vi "MEASURE_hysteresis_multiple_SHG gate_pmt-final.vi"() -> ()   [LabVIEW 2020]
uses:
  <vilib>/DAQmx/read.llb/DAQmx Read.vi
  <vilib>/DAQmx/read.llb/DAQmx Read (Counter U32 1Chan 1Samp).vi
  <vilib>/Analysis/baseanly.llb/Mean (DBL).vi
  <vilib>/DAQmx/create/channels.llb/DAQmx Create Channel (CI-Count Edges).vi
  <instrlib>/Keithley 24XX/Public/Data/Read (Multiple Points).vi
  <vilib>/DAQmx/miscellaneous.llb/DAQmx Fill In Error Info.vi
  <vilib>/Utility/file.llb/Write To Spreadsheet File (DBL).vi
  <instrlib>/Stanford Research 830/Stanford Research 830.lvlib
  <instrlib>/Keithley 2450/Keithley 2450.lvlib
  <resource>/objmgr/daqmx.rc
  <instrlib>/Keithley 24XX/Keithley 24XX.lvlib
  <vilib>/Analysis/NI_AALBase.lvlib
panel:
  in  "topgate-off set":dbl=-5.0
  in  "0ff set{T}/no off set[F]":bool
  out "XY Graph 4":cluster{dbl[], dbl[]}(graph)
  out "XY Graph 3":cluster{dbl[], dbl[]}(graph)
  out "back gate leaking":dbl=2.469318360898143e-10
  out "top gate voltage":dbl format="%#_13g"
  in  "Compliance  Level (1uA)":dbl=1.9999999995789155e-07
  in  "Source Mode  (0: Voltage)":u16(ring) items=["Voltage", "Current"]
  in  "Serial Configuration":T1={"Baud Rate"=9600, "Parity"=0, "Data Bits"=8, "Stop Bits"=10, "Flow Control"=0} {"Flow Control" items=["None", "XON/XOFF", "RTS/CTS", "XON/XOFF & RTS/CTS", "DTR/DSR", "XON/XOFF & DTR/DSR"]; "Stop Bits" items=["1.0"=10, "1.5"=15, "2.0"=20]; "Data Bits" items=["7"=7, "8"=8]; "Parity" items=["None", "Odd", "Even", "Mark", "Space"]; "Baud Rate" items=["300"=300, "600"=600, "1200"=1200, "2400"=2400, "4800"=4800, "9600"=9600, "19200"=19200]}
  in  "back gate address":refnum<visa-resource-name>="GPIB0::25::INSTR"
  in  "top gate thickness":dbl=10.0
  in  "back gate thickness":dbl=30.0
  in  "pure field (T)/pure doping (F)":bool
  in  "Clear Plot 2":bool
  out "XY Graph 2":cluster{dbl[], dbl[]}(graph)
  in  "accumulation":i32=80
  out "Waveform Chart 3":dbl[](graph)=[376.0, 339.0, 337.0, 347.0, 368.0, 343.0, 313.0, 342.0, 356.0, 353.0, 315.0, 360.0, 375.0, 301.0, 363.0, 324.0, 334.0, 324.0, 318.0, 329.0, 312.0, 341.0, 352.0, 336.0, 351.0, 312.0, 361.0, 339.0, 352.0, 315.0, 360.0, 366.0, 324.0, 343.0, 343.0, 330.0, 340.0, 327.0, 393.0, 330.0, 335.0, 353.0, 360.0, 347.0, 337.0, 336.0, 312.0, 331.0, 326.0, 350.0, 344.0, 328.0, 357.0, 355.0, 356.0, 331.0, 328.0, 340.0, 355.0, 387.0, 371.0, 360.0, 331.0, 339.0, 344.0, 367.0, 343.0, 360.0, 360.0, 370.0, 335.0, 366.0, 323.0, 378.0, 373.0, 358.0]
  out "Numeric":dbl=344.60526315789474
  in  "Counter Channel":tag="/Dev1/PFI0"
  in  "error in":errorcluster
  out "loop run":i32=2
  in  "loop #":i32=2
  in  "Save data or not":bool=TRUE
  in  "path (folder + filename)":string="C:\\Users\\User\\Data\\Jason\\03282019\\ pure_bottom_high_6v_rato3 with light2"
  in  "Clear Plot":bool
  out "LOCKIN Measurement":dbl=0.9110010000000001
  in  "Parameter (1: X)":u16(ring)=1 items=["X"=1, "Y"=2, "R"=3, "Theta"=4, "Channel 1"=5, "Channel 2"=6, "Aux In 1"=7, "Aux In 2"=8, "Aux In 3"=9, "Aux In 4"=10]
  out "back gate voltage":dbl format="%#_13g"
  out "top gate leaking":string="-9.306248E-12\n"
  in  "GATE STEP(mv)":i32=450
  in  "GATE Low Value (default 0)":dbl
  in  "GATE High Value":dbl=18.0
  in  "Function (0: Volts) 2":u16(ring) items=["Volts", "Current", "Resistance"]
  in  "Source Compaliance":dbl=1.000000000000001e-07
  in  "topgate address":refnum<visa-resource-name>="GPIB0::18::INSTR"
  in  "SD stabilization(S) 2":dbl=0.1 format="%#_13g"
  in  "Sine Output Amplitude (1 V) 2":dbl=0.05
  in  "GATE / SD stablization 3":dbl=0.1 format="%#_13g"
  in  "frequency":dbl=50.0 format="%#_13g"
  in  "Input Connection (0: Single-Ended Voltage)":u16(ring) items=["Single-Ended Voltage", "Differential Voltage", "1 MOhm Current Gain", "100 MOhm Current Gain"]
  in  "LOCKIN address":refnum<visa-resource-name>="GPIB0::8::INSTR"
  # "Gate2401(top) Setting"
  # "Lock-in"
  # "Gate2450(back) Setting"
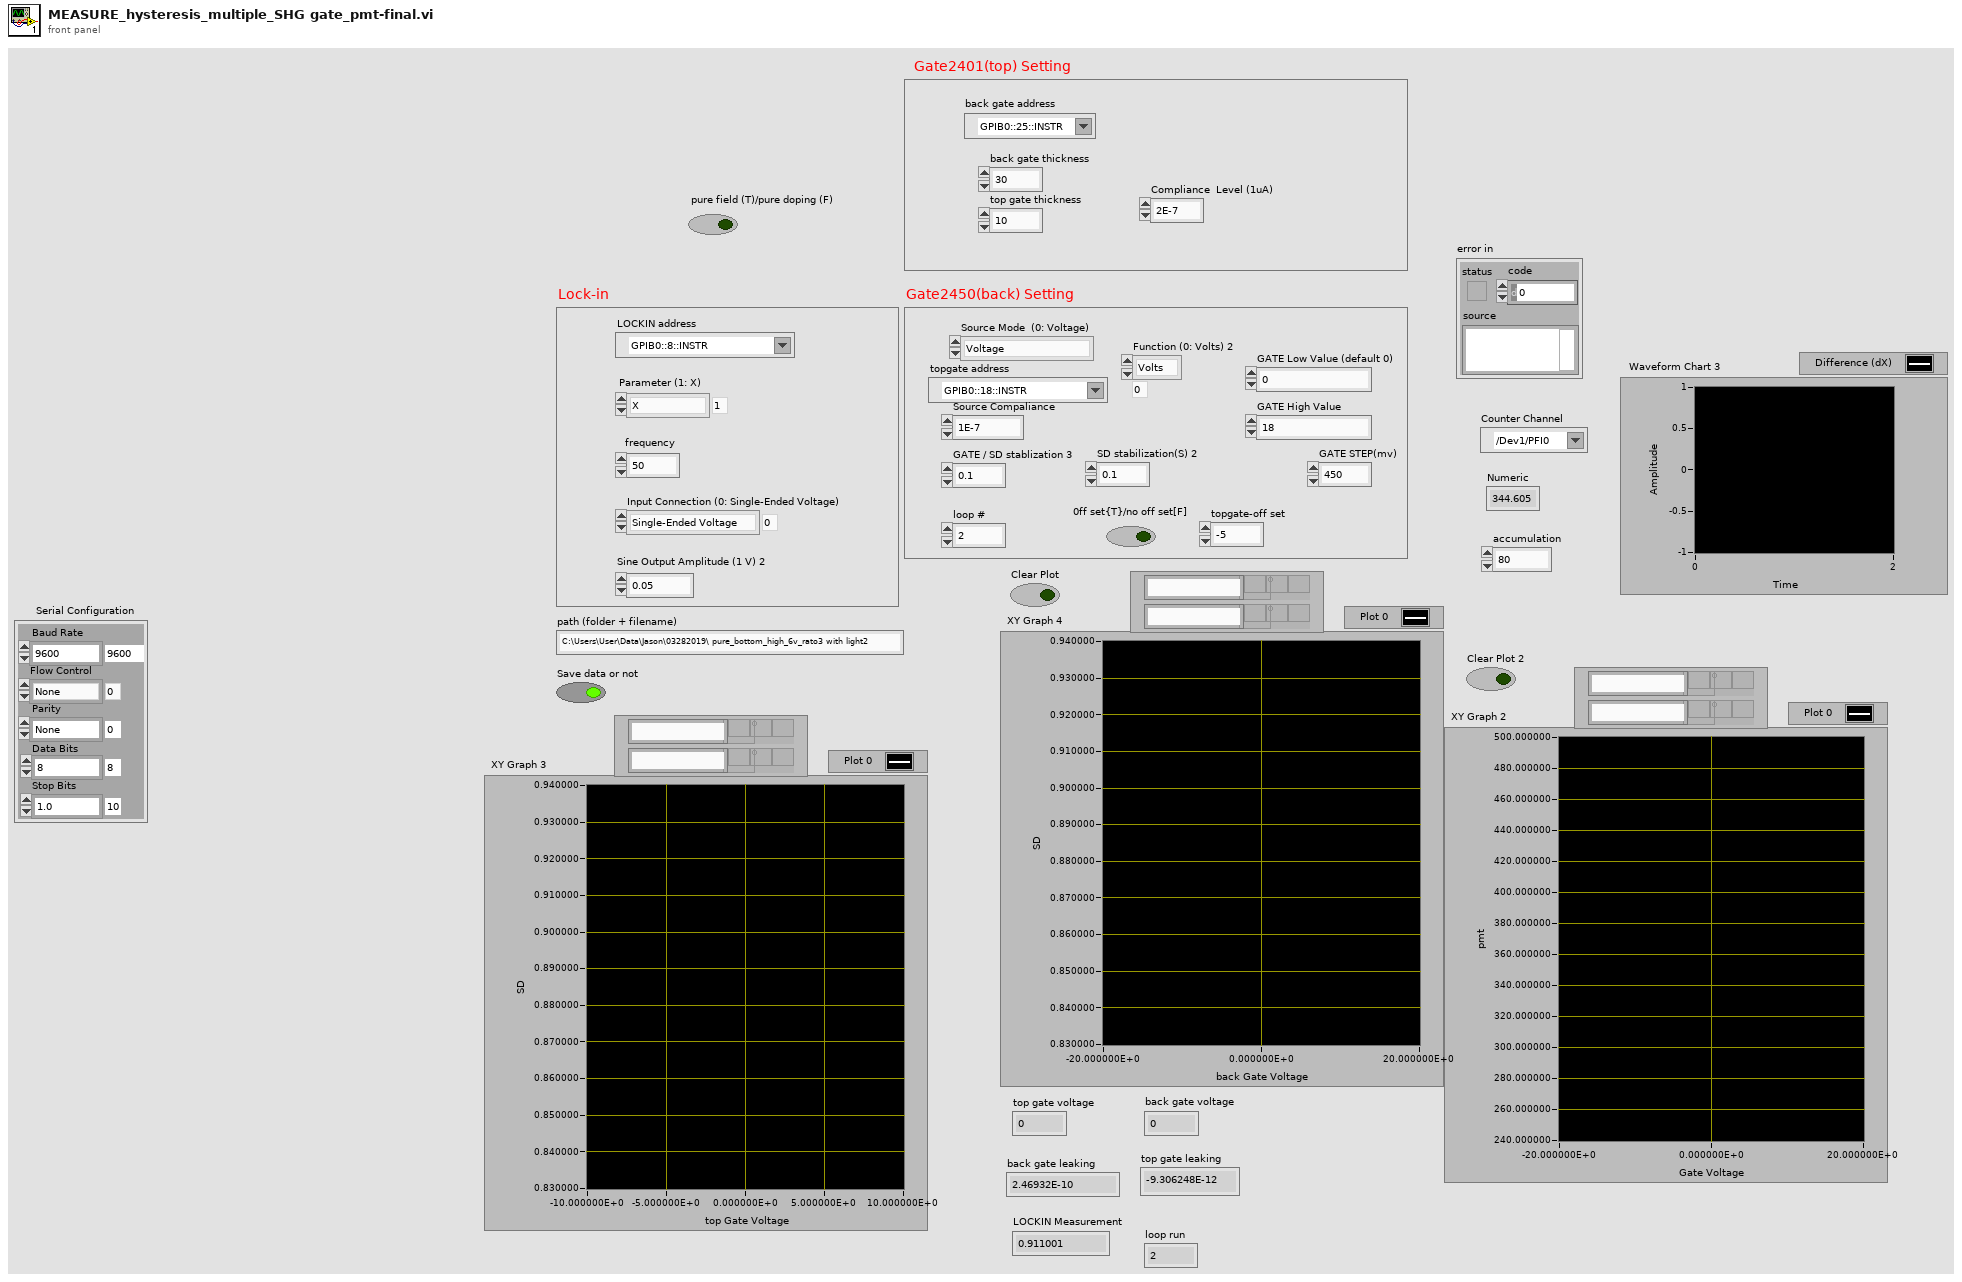
[diagram p1: front panel]
types:
  T1 = cluster{"Baud Rate":u32, "Parity":u16, "Data Bits":u16, "Stop Bits":u16, "Flow Control":u16}
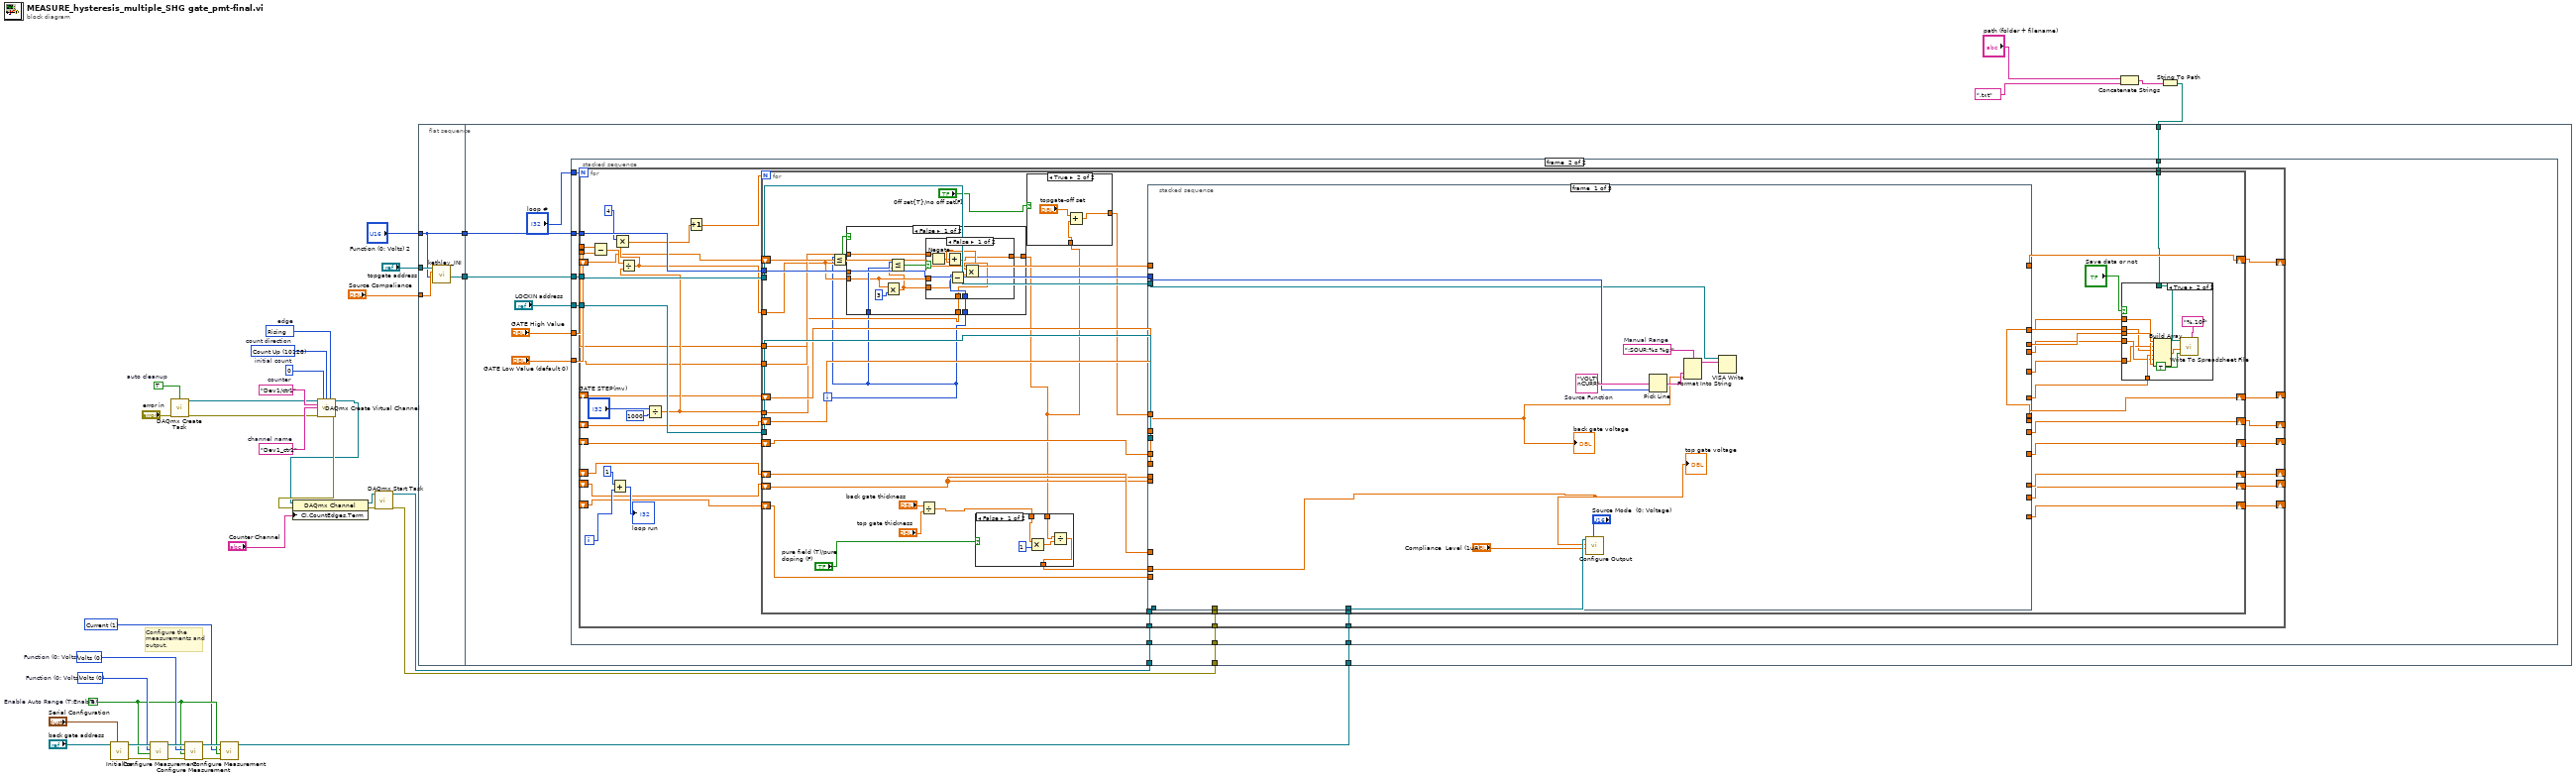
[diagram p0: block diagram]
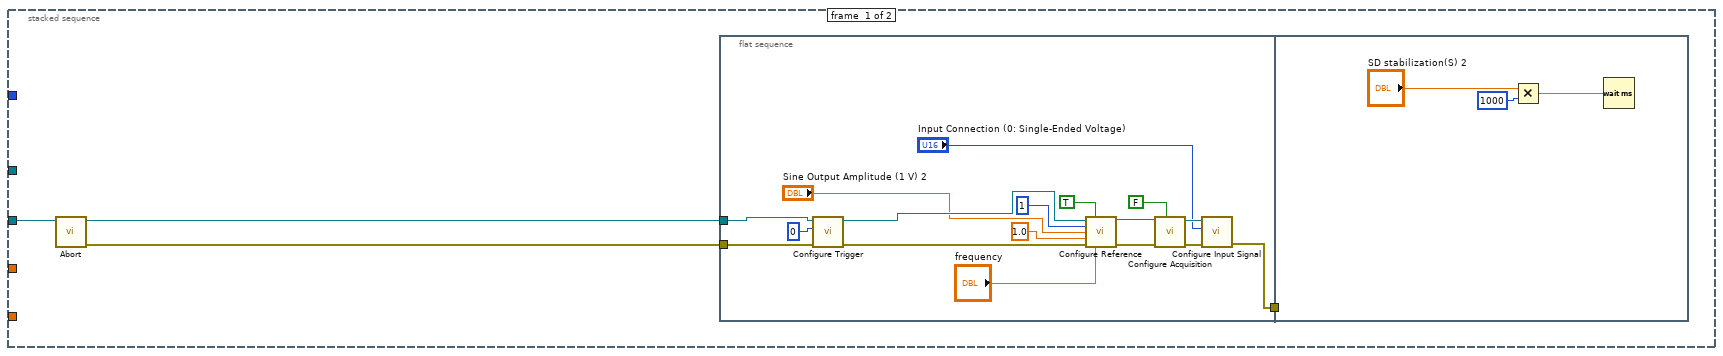
[diagram p2: hidden frame]
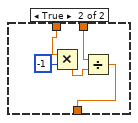
[diagram p4: hidden frame]
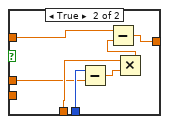
[diagram p6: hidden frame]
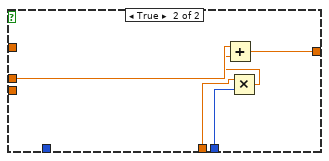
[diagram p7: hidden frame]
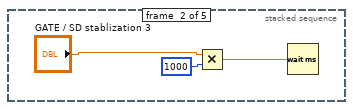
[diagram p8: hidden frame]
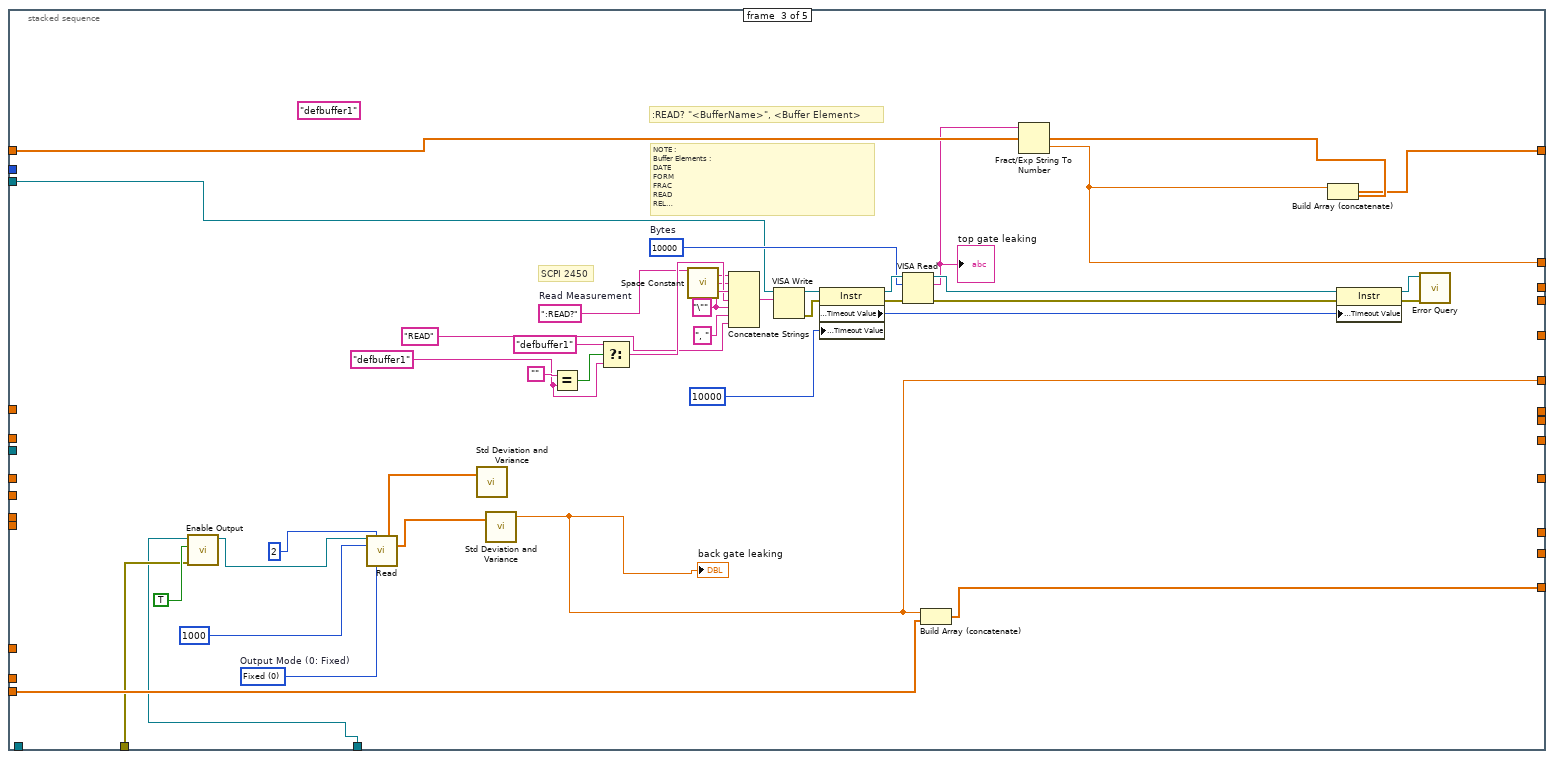
[diagram p9: hidden frame]
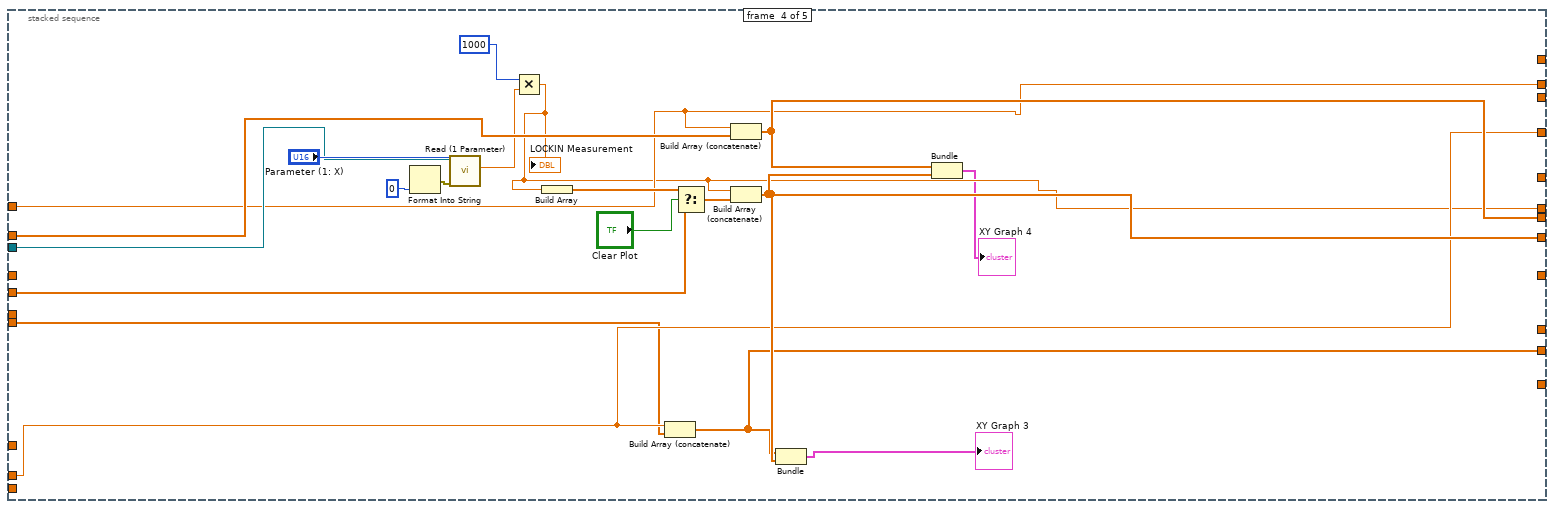
[diagram p10: hidden frame]
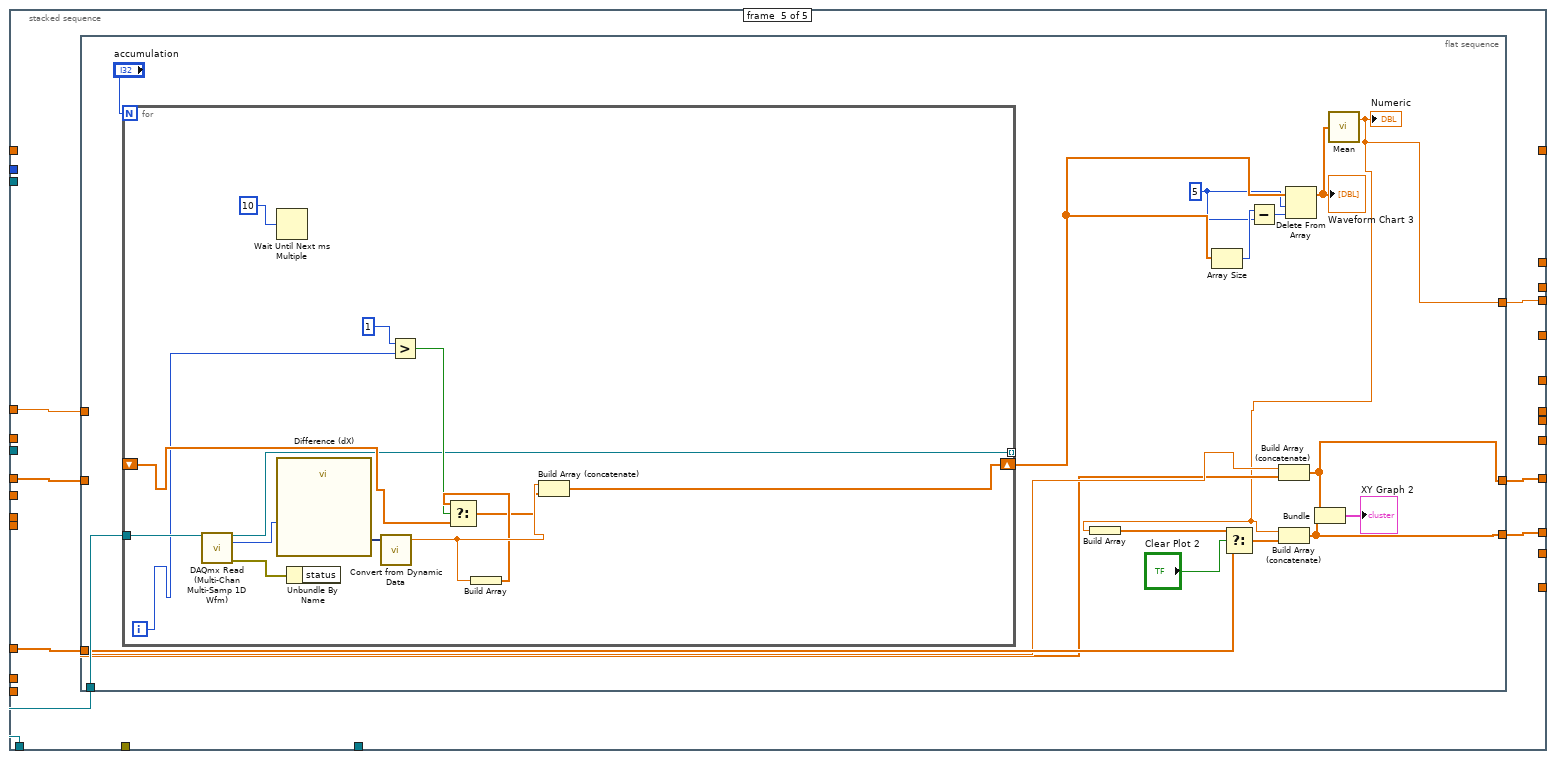
[diagram p11: hidden frame]
diagram:
  w3 = u16 1 items=["Volts", "Current", "Resistance"] ("Function (0: Volts)")
  w4 = TRUE  # Enable Auto Range (T:Enable)
  w7 = u16 0 items=["Volts", "Current", "Resistance"]  # Function (0: Volts)
  w8 = u16 0 items=["Volts", "Current", "Resistance"]  # Function (0: Volts)
  w27 = 10280 items=["Rising"=10280, "Falling"=10171]  # edge
  w26 = 10128 items=["Count Up"=10128, "Count Down"=10124, "Externally Controlled"=10326]  # count direction
  w25 = u32 0  # initial count
  w24 = "Dev1_ctr1"  # channel name
  w23 = "Dev1/ctr1"  # counter
  w21 = TRUE  # auto cleanup
  # "Configure the measurements and output."
  n1 = call <instrlib>:"Initialize.vi"("Serial Configuration"="Serial Configuration", "VISA resource name"="back gate address") -> ("error out"=w13:errorcluster, "VISA resource name out"=w14:refnum<visa-resource-name>)  [unwired: 8 in]
  n2 = call <instrlib>:"Configure Measurement.vi"("error in (no error)"=w13, "Enable Auto Range (T:Enable)"=w4, "Function (0: Volts)"=w8, "VISA resource name"=w14) -> ("error out"=w12:errorcluster, "VISA resource name out"=w11:refnum<visa-resource-name>)  [unwired: 6 in]
  n3 = call <vilib>:"DAQmx Create Task.vi"("auto cleanup"=w21, "error in"="error in") -> ("task out"=w22:refnum<k21>, "error out"=w20:errorcluster)  [unwired: 12 in]
  n4 = call <instrlib>:"Configure Measurement.vi"("error in (no error)"=w12, "Enable Auto Range (T:Enable)"=w4, "Function (0: Volts)"=w7, "VISA resource name"=w11) -> ("error out"=w5:errorcluster, "VISA resource name out"=w6:refnum<visa-resource-name>)  [unwired: 6 in]
  n5 = call <instrlib>:"Configure Measurement.vi"("error in (no error)"=w5, "Enable Auto Range (T:Enable)"=w4, "Function (0: Volts)"=w3, "VISA resource name"=w6) -> ("VISA resource name out"=w2:refnum<visa-resource-name>)  [unwired: 6 in, 1 out]
  n6 = call-poly <vilib>:"DAQmx Create Virtual Channel.vi"("task in"=w22, "initial count"=w25, "count direction"=w26, "edge"=w27, "counter"=w23, "name to assign"=w24, "error in"=w20) -> ("task out"=w28:refnum<k21>, "error out"=w29:errorcluster)  [unwired: 7 in]
  n7 = property class="DAQmx Channel"(reference=w28, error in=w29, "CI.CountEdges.Term"="Counter Channel") -> (reference out=w16:refnum<k21>, error out=w17:errorcluster)
  n8 = call <vilib>:"DAQmx Start Task.vi"("task/channels in"=w16, "error in"=w17) -> ("task out"=w15:refnum<k21>, "error out"=w1:errorcluster)  [unwired: 12 in]
  n9 = flat-sequence {
    tunnel: "topgate address" -> [w42]
    tunnel: "Source Compaliance" -> [w41]
    tunnel: "Function (0: Volts) 2" -> [w39]
    tunnel: [w40] -> w35
    tunnel: [w39] -> w34
    tunnel: w35 -> [w51]
    tunnel: w34 -> [w50]
    tunnel: w30 -> [w47]
    tunnel: w15 -> [w45]
    tunnel: w2 -> [w44]
    tunnel: w1 -> [w43]
    frame #0 {
      n10 = call "kethley_INI.vi"("Function (0: Volts) in"=w39, "Source Compaliance"=w41, "VISA Refnum in"=w42) -> ("VISA resource name out"=w40:refnum<visa-resource-name>)  [unwired: 8 in]
    }
    frame #1 {
      n11 = stacked-sequence {
        tunnel: "LOCKIN address" -> [w55 w84]
        tunnel: w51 -> [_ w85]
        tunnel: w50 -> [_ w86]
        tunnel: "GATE High Value" -> [_ w82]
        tunnel: "GATE Low Value (default 0)" -> [_ w83]
        tunnel: w47 -> [_ w81]
        tunnel: "loop #" -> [_ w80]
        tunnel: w45 -> [_ w79]
        tunnel: w44 -> [_ w78]
        tunnel: w43 -> [_ w77]
        frame #0 {
          n12 = call <instrlib>:"Abort.vi"("VISA resource name"=w55) -> ("error out"=w53:errorcluster, "VISA resource name out"=w54:refnum<visa-resource-name>)  [unwired: 9 in]
          n13 = flat-sequence {
            tunnel: w54 -> [w73]
            tunnel: [w58] -> w56
            tunnel: w53 -> [w57]
            tunnel: w56 -> [_]
            frame #0 {
              n14 = call <instrlib>:"Configure Trigger.vi"("error in (no error)"=w57, "Trigger Source (0: Internal)"=0, "VISA resource name"=w73) -> ("error out"=w67:errorcluster, "VISA resource name out"=w68:refnum<visa-resource-name>)  [unwired: 7 in]
              n15 = call <instrlib>:"Configure Reference.vi"("VISA resource name"=w68, "Auto Phase (T: Enabled)"=TRUE, "Reference Source (1: Internal)"=1, "Sine Output Amplitude (1 V)"="Sine Output Amplitude (1 V) 2", "Detection Harmonic Number (1)"=1.0 ("output voltage 2"), "error in (no error)"=w67, "Internal Reference Frequency (1000 Hz)"="frequency") -> ("VISA resource name out"=w65:refnum<visa-resource-name>, "error out"=w60:errorcluster)  [unwired: 7 in]
              n16 = call <instrlib>:"Configure Acquisition.vi"("Continuous Storage (T: Enable)"=FALSE, "error in (no error)"=w60, "VISA resource name"=w65) -> ("error out"=w59:errorcluster, "VISA resource name out"=w63:refnum<visa-resource-name>)  [unwired: 7 in]
              n17 = call <instrlib>:"Configure Input Signal.vi"("error in (no error)"=w59, "Input Connection (0: Single-Ended Voltage)"="Input Connection (0: Single-Ended Voltage)", "VISA resource name"=w63) -> ("error out"=w58:errorcluster)  [unwired: 7 in, 1 out]
            }
            frame #1 {
              n18 = Multiply(x="SD stabilization(S) 2", y=1000) -> (x*y=w76:dbl)
              n19 = Wait (ms)(milliseconds to wait=w76) -> ()  [unwired: 1 out]
            }
          }
        }
        frame #1 {
          n20 = for {
            N: w80 -> [_]
            tunnel: w86 -> [w120]
            tunnel: w85 -> [w119]
            tunnel: w84 -> [w118]
            tunnel: w83 -> [w112]
            tunnel: w82 -> [w111]
            tunnel: w81 -> [w110]
            shift-right: [w106] -> _
            shift-left: _ -> [w105]
            shift-right: [w104] -> _
            shift-left: _ -> [w102]
            shift-right: [w103] -> _
            shift-left: _ -> [w101]
            tunnel: w79 -> [w97]
            shift-right: [w96] -> _
            shift-left: _ -> [w95]
            shift-right: [w94] -> _
            shift-left: _ -> [w93]
            shift-right: [w92] -> _
            shift-left: _ -> [w91]
            shift-right: [w90] -> _
            shift-left: _ -> [w89]
            tunnel: w78 -> [w88]
            tunnel: w77 -> [w87]
            i -> [w99]
            n21 = Subtract(x=w111, y=w112) -> (x-y=w114:dbl)
            n22 = Add(x=1, y=w99) -> (x+y=→"loop run":i32)
            n23 = Divide(x="GATE STEP(mv)", y=1000) -> (x/y=w113:dbl)
            n24 = Divide(x=w114, y=w113) -> (x/y=w109:dbl)
            n25 = Multiply(x=4, y=w109) -> (x*y=w108:dbl)
            n26 = Increment(x=w108) -> (x+1=w107:dbl)
            n27 = for {
              N: w107 -> [_]
              tunnel: w120 -> [w162]
              tunnel: w119 -> [w161]
              tunnel: w118 -> [w160]
              tunnel: w113 -> [w151]
              shift-right: [w159] -> w106
              shift-left: w105 -> [w158]
              shift-right: [w155] -> w103
              shift-left: w101 -> [w157]
              shift-right: [w154] -> w104
              shift-left: w102 -> [w156]
              tunnel: w109 -> [w149]
              tunnel: w112 -> [w152]
              tunnel: w111 -> [w150]
              tunnel: w110 -> [w144]
              tunnel: w97 -> [w142]
              shift-right: [w141] -> w96
              shift-left: w95 -> [w127]
              shift-right: [w140] -> w94
              shift-left: w93 -> [w139]
              shift-right: [w137] -> w92
              shift-left: w91 -> [w128]
              shift-right: [w136] -> w90
              shift-left: w89 -> [w126]
              tunnel: w88 -> [w134]
              tunnel: w87 -> [w125]
              i -> [w148]
              n28 = Less Or Equal?(x=w148, y=w149) -> (x <= y?=w153:bool)
              n29 = case shown="False" w153 {
                tunnel: w152 -> [_ w215]
                tunnel: w148 -> [w195 w214]
                tunnel: w151 -> [w194 w213]
                tunnel: [w192 w211] -> w122
                tunnel: w150 -> [w193 _]
                tunnel: w149 -> [w188 _]
                tunnel: w148 -> [w191 _]
                frame False {
                  n30 = Multiply(x=w188, y=3) -> (x*y=w187:dbl)
                  n31 = Less Or Equal?(x=w191, y=w187) -> (x <= y?=w189:bool)
                  n32 = case shown="False" w189 {
                    tunnel: w195 -> [w203 w210]
                    tunnel: w194 -> [w201 w208]
                    tunnel: w193 -> [w197 w206]
                    tunnel: [w199 w205] -> w192
                    tunnel: w188 -> [_ w204]
                    tunnel: w187 -> [w196 _]
                    frame False {
                      n33 = Negate(x=w197) -> (-x=w198:dbl)
                      n34 = Subtract(x=w203, y=w196) -> (x-y=w202:dbl)
                      n35 = Multiply(x=w201, y=w202) -> (x*y=w200:dbl)
                      n36 = Add(x=w198, y=w200) -> (x+y=w199:dbl)
                    }
                    frame True {
                      n37 = Subtract(x=w210, y=w204) -> (x-y=w209:dbl)
                      n38 = Multiply(x=w208, y=w209) -> (x*y=w207:dbl)
                      n39 = Subtract(x=w206, y=w207) -> (x-y=w205:dbl)
                    }
                  }
                }
                frame True {
                  n40 = Multiply(x=w213, y=w214) -> (x*y=w212:dbl)
                  n41 = Add(x=w215, y=w212) -> (x+y=w211:dbl)
                }
              }
              n42 = Divide(x="back gate thickness", y="top gate thickness") -> (x/y=w133:dbl)
              n43 = case shown="False" "pure field (T)/pure doping (F)" {
                tunnel: w133 -> [w170 w176]
                tunnel: [w167 w174] -> w129
                tunnel: w122 -> [w168 w173]
                frame False {
                  n44 = Multiply(x=w170, y=1) -> (x*y=w169:dbl)
                  n45 = Divide(x=w168, y=w169) -> (x/y=w167:dbl)
                }
                frame True {
                  n46 = Multiply(x=w176, y=-1) -> (x*y=w172:dbl)
                  n47 = Divide(x=w173, y=w172) -> (x/y=w174:dbl)
                }
              }
              n48 = case shown="True" "0ff set{T}/no off set[F]" {
                tunnel: w122 -> [w163 w166]
                tunnel: [w163 w164] -> w121
                frame False {
                }
                frame True {
                  n49 = Add(x="topgate-off set", y=w166) -> (x+y=w164:dbl)
                }
              }
              n50 = stacked-sequence {
                tunnel: w162 -> [w222 _ _ _ _]
                tunnel: w161 -> [w221 _ w246 _ _]
                tunnel: w160 -> [_ _ _ w280 _]
                tunnel: w121 -> [w220 _ _ w279 w291]
                tunnel: [_ _ w244 _ _] -> w159
                tunnel: w158 -> [_ _ w245 _ _]
                tunnel: w157 -> [_ _ _ w283 _]
                tunnel: w156 -> [_ _ _ w281 _]
                tunnel: [_ _ _ w276 _] -> w155
                tunnel: [_ _ _ w282 _] -> w154
                tunnel: [_ _ _ w270 _] -> w147
                tunnel: [_ _ _ w279 _] -> w146
                tunnel: [_ _ w242 _ _] -> w145
                tunnel: w142 -> [_ _ _ _ w295]
                tunnel: [_ _ _ _ w294] -> w141
                tunnel: w127 -> [_ _ _ _ w293]
                tunnel: [_ _ _ _ w292] -> w140
                tunnel: w139 -> [_ _ _ _ w290]
                tunnel: [_ _ _ _ w289] -> w138
                tunnel: [_ _ w236 _ _] -> w137
                tunnel: [_ _ _ w275 _] -> w136
                tunnel: w126 -> [_ _ _ _ _]
                tunnel: [_ _ _ w274 _] -> w135
                tunnel: [_ _ w235 _ _] -> w124
                tunnel: w134 -> [w218 _ w231 _ _]
                tunnel: w129 -> [w216 _ _ w274 _]
                tunnel: w128 -> [_ _ w234 _ _]
                tunnel: w126 -> [_ _ _ w273 _]
                tunnel: w125 -> [_ _ w232 _ _]
                frame #0 {
                  w224 = "VOLT\nCURR"  # Source Function
                  w225 = ":SOUR:%s %g;"  # Manual Range
                  n51 = call <instrlib>:"Configure Output.vi"("Source Mode  (0: Voltage)"="Source Mode  (0: Voltage)", "Compliance  Level (0.1)"="Compliance  Level (1uA)", "Output Level (0)"=w216, "VISA resource name"=w218) -> ()  [unwired: 6 in, 2 out]
                  n52 = Pick Line(multi-line string=w224, line index=w222) -> (output string=w223:string)  [unwired: 1 out]
                  n53 = Format Into String(format string=w225, w223, w220) -> (resulting string=w226:string)  [unwired: 2 in, 1 out]
                  n54 = VISA Write(VISA resource name=w221, write buffer=w226) -> ()  [unwired: 1 in, 3 out]
                  "back gate voltage" <- w220
                  "top gate voltage" <- w216
                }
                frame #1 {
                  n55 = Multiply(x="GATE / SD stablization 3", y=1000) -> (x*y=w229:dbl)
                  n56 = Wait (ms)(milliseconds to wait=w229) -> ()  [unwired: 1 out]
                }
                frame #2 {
                  w239 = u16 0 items=["Fixed", "Sweep", "List"]  # Output Mode (0: Fixed)
                  w257 = "defbuffer1" ("Buffer Name (defbuffer1) 2")
                  (unwired) "defbuffer1" ("t")
                  w255 = "\""
                  w252 = ":READ?"  # Read Measurement
                  w261 = u32 10000  # Bytes
                  # "NOTE :\nBuffer Elements :\nDATE\nFORM\nFRAC\nREAD\nREL\nSEC\nSOUR\nSOURFORM\nSOURSTAT\nSOURUNIT\nSTAT\nTIME\nTsT\nUNIT"
                  # ":READ? \"<BufferName>\", <Buffer Element>"
                  # "SCPI 2450"
                  n57 = call <instrlib>:"Enable Output.vi"("error in (no error)"=w232, "Enable Output (T: Enable)"=TRUE, "VISA resource name"=w231) -> ("VISA resource name out"=w230:refnum<visa-resource-name>)  [unwired: 7 in, 1 out]
                  n58 = call-poly <instrlib>:"Read.vi"("VISA resource name"=w230, "Sample Count (1)"=u32 2 ("Number of Samples"), "Timeout (10000 ms)"=1000, "Output Mode (0: Fixed)"=w239) -> ("Voltage"=w237:sgl[], "Current"=w238:sgl[])  [unwired: 5 in, 5 out]
                  n59 = call <vilib>:"Std Deviation and Variance.vi"("X"=w237) -> ()  [unwired: 1 in, 3 out]
                  n60 = call <vilib>:"Std Deviation and Variance.vi"("X"=w238) -> ("mean"=w235:dbl)  [unwired: 1 in, 2 out]
                  "back gate leaking" <- w235
                  n61 = Equal?(x="", y=w257) -> (x = y?=w258:bool)
                  n62 = Select(t="defbuffer1", s=w258, f=w257) -> (s? t:f=w254:string)
                  n63 = call <vilib>:"Space Constant.vi"() -> ("String"=w253:string)
                  n64 = Concatenate Strings(w252, w253, w255, w254, w255, ", " ("string"), "READ" ("Buffer Elements 2")) -> (w268:string)
                  n65 = VISA Write(VISA resource name=w246, write buffer=w268) -> (VISA resource name out=w260:refnum<visa-resource-name>, error out=w267:errorcluster)  [unwired: 1 in, 1 out]
                  n66 = property class="Instr"(reference=w260, error in=w267, "General Settings:Timeout Value"=10000 ("Timeout (10000 ms) 2")) -> (reference out=w266:refnum<visa-resource-name>, error out=w265:errorcluster, "General Settings:Timeout Value"=w262:u32)
                  n67 = VISA Read(VISA resource name=w266, byte count=w261, error in (no error)=w265) -> (VISA resource name out=w264:refnum<visa-resource-name>, read buffer=w243:string, error out=w263:errorcluster)  [unwired: 1 out]
                  "top gate leaking" <- w243
                  n68 = Build Array (concatenate)(w235, w234) -> (w236:dbl[])
                  n69 = Fract/Exp String To Number(string=w243) -> (number=w242:dbl)  [unwired: 3 in, 1 out]
                  n70 = Build Array (concatenate)(w242, w245) -> (w244:dbl[])
                  n71 = property class="Instr"(reference=w264, error in=w263, "General Settings:Timeout Value"=w262) -> (reference out=w250:refnum<visa-resource-name>, error out=w249:errorcluster)
                  n72 = call <instrlib>:"Error Query.vi"("error in (no error)"=w249, "VISA resource name"=w250) -> ()  [unwired: 10 out]
                }
                frame #3 {
                  n73 = Format Into String(0) -> (error out=w288:errorcluster)  [unwired: 3 in, 1 out]
                  n74 = call <instrlib>:"Read (1 Parameter).vi"("error in (no error)"=w288, "Parameter (1: X)"="Parameter (1: X)", "VISA resource name"=w280) -> ("Measurement"=w271:dbl)  [unwired: 6 in, 2 out]
                  n75 = Multiply(x=1000, y=w271) -> (x*y=w270:dbl)
                  "LOCKIN Measurement" <- w270
                  n76 = Build Array(w270) -> (w286:dbl[])
                  n77 = Build Array (concatenate)(w274, w273) -> (w275:dbl[])
                  n78 = Select(t=w286, s="Clear Plot", f=w283) -> (s? t:f=w278:dbl[])
                  n79 = Build Array (concatenate)(w279, w281) -> (w282:dbl[])
                  n80 = Build Array (concatenate)(w270, w278) -> (w276:dbl[])
                  n81 = Bundle(w275, w276) -> (→"XY Graph 3":cluster{dbl[], dbl[]})  [unwired: 1 in]
                  n82 = Bundle(w282, w276) -> (→"XY Graph 4":cluster{dbl[], dbl[]})  [unwired: 1 in]
                }
                frame #4 {
                  n83 = flat-sequence {
                    tunnel: w295 -> [w307]
                    tunnel: [w300] -> w294
                    tunnel: w293 -> [w301]
                    tunnel: [w299] -> w292
                    tunnel: w291 -> [w298]
                    tunnel: w290 -> [w297]
                    tunnel: [w296] -> w289
                    frame #0 {
                      w309 = 5
                      n84 = for {
                        N: "accumulation" -> [_]
                        tunnel: w307 -> [w317]
                        shift-right: [w316] -> w311
                        shift-left: _ -> [w315]
                        tunnel: [w313] -> _ mode=indexing
                        i -> [w314]
                        n85 = call-poly "DAQmx Read (Multi-Chan Multi-Samp 1D Wfm).vi"("task/channels in"=w317) -> ("task out"=w313:refnum<k21>, "data"=w323:u32, "error out"=w324:errorcluster)  [unwired: 12 in]
                        n86 = Wait Until Next ms Multiple(millisecond multiple=10) -> ()  [unwired: 1 out]
                        n87 = call "Difference (dX)"("Signals"=w323) -> ("Result"=w326:dynamicdata)  [unwired: 5 in, 1 out]
                        n88 = Unbundle By Name(w324) -> ()  [unwired: 1 out]
                        n89 = call "Convert from Dynamic Data"("Dynamic Data Type"=w326) -> ("Scalar"=w322:dbl)  [unwired: 3 in]
                        n90 = Greater?(x=1, y=w314) -> (0:w318:bool)
                        n91 = Build Array(w322) -> (w321:dbl[])
                        n92 = Select(t=w321, s=w318, f=w315) -> (s? t:f=w320:dbl[])
                        n93 = Build Array (concatenate)(w322, w320) -> (w316:dbl[])
                      }
                      n94 = Array Size(array=w311) -> (size(s)=w310:i32)
                      n95 = Subtract(x=w310, y=w309) -> (x-y=w308:i32)
                      n96 = Build Array (concatenate)(w298, w297) -> (w299:dbl[])
                      n97 = Delete From Array(array=w311, length=w309, index=w308) -> (array with subset deleted=w306:dbl[])  [unwired: 1 out]
                      "Waveform Chart 3" <- w306
                      n98 = call-poly <vilib>:"Mean.vi"("X"=w306) -> ("mean"=w296:dbl)  [unwired: 1 out]
                      "Numeric" <- w296
                      n99 = Build Array(w296) -> (w304:dbl[])
                      n100 = Select(t=w304, s="Clear Plot 2", f=w301) -> (s? t:f=w305:dbl[])
                      n101 = Build Array (concatenate)(w296, w305) -> (w300:dbl[])
                      n102 = Bundle(w299, w300) -> (→"XY Graph 2":cluster{dbl[], dbl[]})  [unwired: 1 in]
                    }
                  }
                }
              }
              n103 = case shown="True" "Save data or not" {
                tunnel: w147 -> [_ w177]
                tunnel: w146 -> [_ w186]
                tunnel: w145 -> [_ w185]
                tunnel: w144 -> [_ w183]
                tunnel: w138 -> [_ w179]
                tunnel: w135 -> [_ w178]
                tunnel: w124 -> [_ w180]
                frame False {
                }
                frame True {
                  n104 = Build Array(w186, w178, w177, w180, w179, w185) -> (w184:dbl[])
                  n105 = call-poly <vilib>:"Write To Spreadsheet File.vi"("format (%.3f)"="%.10f", "append to file? (new file:F)"=TRUE, "1D data"=w184, "file path (dialog if empty)"=w183) -> ()  [unwired: 4 in, 1 out]
                }
              }
            }
          }
        }
      }
    }
  }
  n106 = Concatenate Strings("path (folder + filename)", ".txt") -> (w31:string)
  n107 = String To Path(string=w31) -> (path=w30:path)
